vi "PASSFAIL.vi"(11 "E":bool) -> (3 "S":string)   [LabVIEW 2020]
doc: "S = ( E ) ? PASS : FAIL ;"
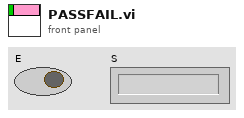
[diagram p1: front panel]
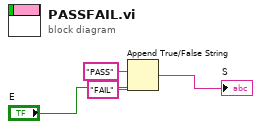
[diagram p0: block diagram]
diagram:
  n1 = Append True/False String(1:"E", 2:"FAIL" ("chaîne faux"), 3:"PASS" ("chaîne vrai")) -> (0:→"S":string)  [unwired: 1 in]
